vi "Format_group_name.vi"(11 "Include \nDate":bool) -> (3 "Group name":string)   [LabVIEW 2015]
uses:
  MARS_Global_var.vi
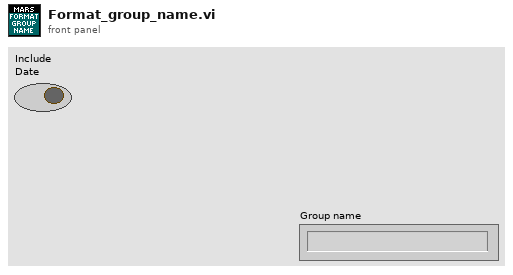
[diagram p1: front panel]
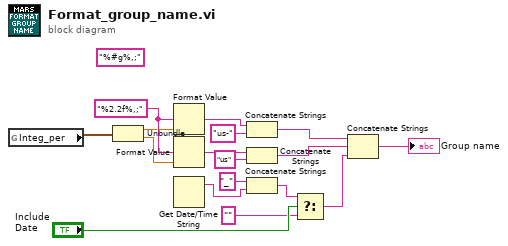
[diagram p0: block diagram]
diagram:
  (unwired) "%#g%,;" ("format string")
  w6 = "%2.2f%,;" ("format string")
  n1 = global read "MARS_Global_var.vi" "Integ_per"() -> (w2:cluster{dbl, dbl})
  n2 = Unbundle(w2) -> (w4:dbl, w5:dbl)
  n3 = Format Value(format string=w6, value (0)=w4) -> (output string=w7:string)  [unwired: 1 in]
  n4 = Format Value(format string=w6, value (0)=w5) -> (output string=w8:string)  [unwired: 1 in]
  n5 = Get Date/Time String() -> (date string=w1:string)  [unwired: 3 in, 1 out]
  n6 = Concatenate Strings(w7, "us-" ("string")) -> (w10:string)
  n7 = Concatenate Strings(w8, "us" ("string")) -> (w11:string)
  n8 = Concatenate Strings("_" ("string"), w1) -> (w17:string)
  n9 = Select(t=w17, s="Include \nDate", f="") -> (s? t:f=w15:string)
  n10 = Concatenate Strings(w10, w11, w15) -> (→"Group name":string)
